vi "Test View get View VI Reference.vi"(8 "error in (no error)":errorcluster, 11 "View Test In":refnum<class "View Test.lvclass">) -> (0 "error out":errorcluster, 3 "View Test Out":refnum<class "View Test.lvclass">)   [LabVIEW 2020, in "View Test.lvclass"]
uses:
  View Test.lvclass
  C:/Program Files (x86)/National Instruments/LabVIEW 2020/vi.lib/Astemes/LUnit/Test Case.lvclass
  Framework/Process/Process.lvclass/Process.ctl
  Framework/View/View.lvclass/View.ctl
  <vilib>/Astemes/LUnit/Test Case.lvclass/Test Case.ctl
  3d873725-d398-442b-bc29-af08f8813fb5.vi
  Framework/Process/Protected/Messaging/Request Message.vi
  Framework/Process/Public/Lifecycle/Get Lifecycle State.vi
  <vilib>/Astemes/LUnit/Palette/Pass.vi
  <vilib>/Astemes/LUnit/Palette/Fail.vi
  <vilib>/Astemes/LUnit/Set Assertion Type.vi
  Framework/Process/Private/SubVIs/Wait for finish.vi
  Framework/Process/Private/SubVIs/Set Lifecycle State.vi
  Framework/Process/Protected/Messaging/Send Message.vi
  <vilib>/Astemes/LUnit/Compare Variants.vi
  <vilib>/Astemes/LUnit/Describe Comparison.vi
  Framework/Process/Private/SubVIs/Handle Debug Data.vi
  Framework/Process/Private/SubVIs/Enqueue Request Message.vi
  <vilib>/Utility/error.llb/Clear Errors.vi
  <vilib>/Astemes/LUnit/Add test result.vi
  <vilib>/Astemes/LUnit/Variant to string.vi
  Framework/Logging/Log Debug.vi
  <vilib>/AdvancedString/1D String Array to Delimited String.vi
  <vilib>/Utility/High Resolution Relative Seconds.vi
  <vilib>/Astemes/LUnit/LUnit Record Assertion Result.vi
  <vilib>/Astemes/LUnit/LUnit Aggregate Assertion Results.vi
  <vilib>/Astemes/LUnit/Method Result/LUnit Merge Status.vi
  <vilib>/Astemes/LUnit/LUnit Concatenate result strings.vi
  Framework/View/View.lvclass
  C:/Git/astemes-triarc-framework/source/Framework/Process/Process.lvclass
  <vilib>/Utility/error.llb/Error Cluster From Error Code.vi
  Framework/Process/Public/Read Name.vi
  Framework/Process/Private/SubVIs/Wait for Response Message.vi
  <vilib>/Utility/Data Type/Get Type Information.vi
  <vilib>/Utility/LVClass/Get LV Class Name.vi
  Framework/Process/Process.lvclass
  View Test.lvclass/View Test.ctl
  <vilib>/Astemes/LUnit/Test Case.lvclass
  C:/Git/astemes-triarc-framework/source/Framework/Base/Base.lvclass
  C:/Git/astemes-triarc-framework/source/Framework/Error Handler Interface/Error Handler Interface.lvclass
  C:/Git/astemes-triarc-framework/source/Framework/Logging/Logging.lvclass
  C:/Git/astemes-triarc-framework/source/Framework/View/View.lvclass
  C:/Git/astemes-triarc-framework/source/Framework Test Suite/Process Test/Process Test.lvclass
  C:/Git/astemes-triarc-framework/source/Framework Test Suite/Base Class Test/Base Test.lvclass
  C:/Git/astemes-triarc-framework/source/Framework Test Suite/View Test/View Test.lvclass
  Process Test/Process Test.lvclass
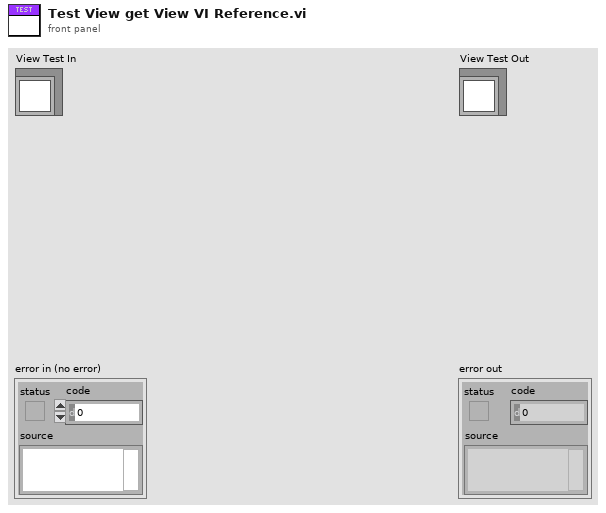
[diagram p1: front panel]
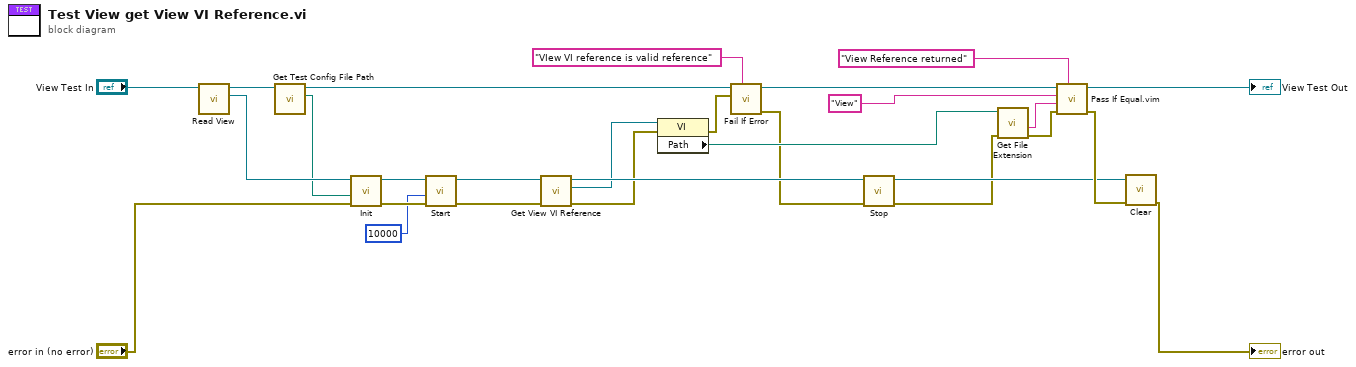
[diagram p0: block diagram]
diagram:
  n1 = call "Read View.vi"("View Test In"="View Test In") -> ("View"=w27:refnum<class "View.lvclass">, "View Test Out"=w28:refnum<class "View Test.lvclass">)  [unwired: 8 in, 1 out]
  n2 = call "Get Test Config File Path.vi"("Process Test In"=w28) -> ("Test config path"=w1:path, "Process Test Out"=w2:refnum<class "View Test.lvclass">)  [unwired: 8 in, 1 out]
  n3 = call-dynamic "Init.vi"("error in (no error)"="error in (no error)", "Config File Path"=w1, "View In"=w27) -> ("error out"=w19:errorcluster, "View Out"=w20:refnum<class "View.lvclass">)  [unwired: 7 in]
  n4 = call "Start.vi"("error in (no error)"=w19, "Timeout [ms] (-1)"=10000, "Process In"=w20) -> ("error out"=w14:errorcluster, "Process Out"=w15:refnum<class "View.lvclass">)  [unwired: 6 in, 1 out]
  n5 = call "Get View VI Reference.vi"("error in (no error)"=w14, "View In"=w15) -> ("error out"=w7:errorcluster, "View VI Reference"=w13:refnum<vi>, "View Out"=w18:refnum<class "View.lvclass">)  [unwired: 7 in]
  n6 = property class="VI"(reference=w13, error in=w7) -> (error out=w6:errorcluster, "Path"=w12:path)  [unwired: 1 out]
  n7 = call <vilib>:"Fail If Error.vi"("Description"="VIew VI reference is valid reference", "Assert error"=w6, "LUnit Test Case In"=w2) -> ("error out"=w4:errorcluster, "LUnit Test Case Out"=w8:refnum<class "View Test.lvclass">)  [unwired: 7 in]
  n8 = call "Stop.vi"("error in (no error)"=w4, "Process In"=w18) -> ("error out"=w16:errorcluster, "Process Out"=w17:refnum<class "View.lvclass">)  [unwired: 7 in, 1 out]
  n9 = call <vilib>:"Get File Extension.vi"("error in (no error)"=w16, "file"=w12) -> ("error out"=w9:errorcluster, "filename without extension"=w11:string)  [unwired: 5 in, 3 out]
  n10 = call "Pass If Equal.vim"("Description"="View Reference returned", "error in (no error)"=w9, "Actual"=w11, "Expected"="View", "LUnit Test Case In"=w8) -> ("error out"=w26:errorcluster, "LUnit Test Case Out"=→"View Test Out":refnum<class "View Test.lvclass">)  [unwired: 5 in]
  n11 = call-dynamic "Clear.vi"("error in (no error)"=w26, "View In"=w17) -> ("error out"=→"error out":errorcluster)  [unwired: 9 in]
